vi "Build Qualified Name.vi"(3 "name":string, 5 "base name":string) -> (1 "appended name":string)   [LabVIEW 2020, in "MeasurementService Editor.lvlib"]
uses:
  MeasurementService Editor.lvlib
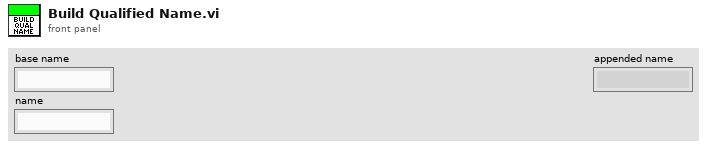
[diagram p1: front panel]
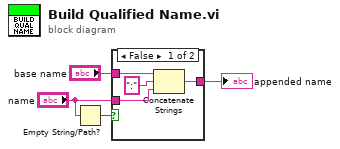
[diagram p0: block diagram]
diagram:
  n1 = Empty String/Path?(string/path="name") -> (empty?=w1:bool)
  n2 = case shown="False" w1 {
    tunnel: "base name" -> [w7 w9]
    tunnel: [w6 w9] -> w3
    tunnel: "name" -> [w5 _]
    frame False {
      n3 = Concatenate Strings(w7, ":" ("string"), w5) -> (w6:string)
    }
    frame True {
    }
  }
  "appended name" <- w3
